vi "Get Variant Data Size.vi"(8 "error in (no error)":errorcluster, 10 "Data String":u8[](array[numeric]), 11 "Type Descriptor":i16[](array[numeric])) -> (0 "error out":errorcluster, 2 "Data Size":i32)   [LabVIEW 2017, in "Composition.lvlib"]
doc: "Gets the data size of a boxed variant."
uses:
  Composition.lvlib
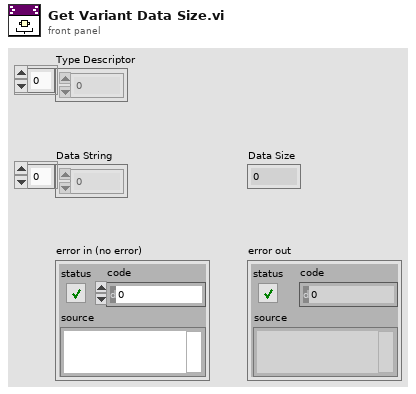
[diagram p1: front panel]
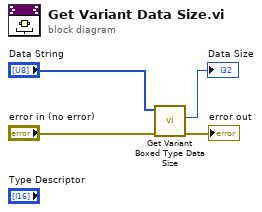
[diagram p0: block diagram]
diagram:
  n1 = call "Get Variant Boxed Type Data Size.vi"("error in (no error)"="error in (no error)", "Data String"="Data String") -> ("error out"=→"error out":errorcluster, "Data Size"=→"Data Size":i32)  [unwired: 7 in, 1 out]
